vi "read e-series file names.vi"(8 "error in (no error)":errorcluster, 11 "INI File":string) -> (0 "error out":errorcluster, 3 "E-Series File Names":T1)   [LabVIEW 2018, in "E-Series Reader.lvlib"]
doc: "Reads the file names of the E-series from the INI configuration file.\n\nReads an INI configuration file and retrieves the file names associated with the E-series. The VI iterates through the sections defined in the configuration file, retrieves the keys, and reads the value of the <b>Filename</b> key from each section. Returns an array of file names for subsequent loading by <b>Read E Series.vi</b>."
uses:
  E-Series Reader/E-Series Reader.lvlib
  E-Series Reader/E-Series File Names--array.ctl
  <vilib>/Utility/config.llb/Read Key (String).vi
  <vilib>/Utility/config.llb/NI_LVConfig.lvlib
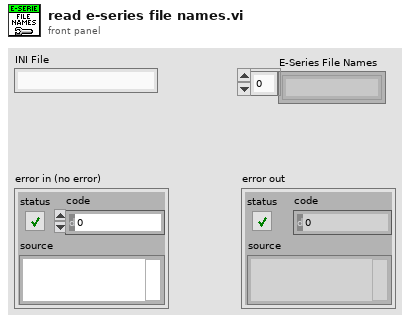
[diagram p1: front panel]
types:
  T1 = typedef "E-Series Reader.lvlib/E-Series File Names--array.ctl" = string[]
  T2 = typedef "NI_LVConfig.lvlib/Config Data RefNum.ctl" = refnum<k1>
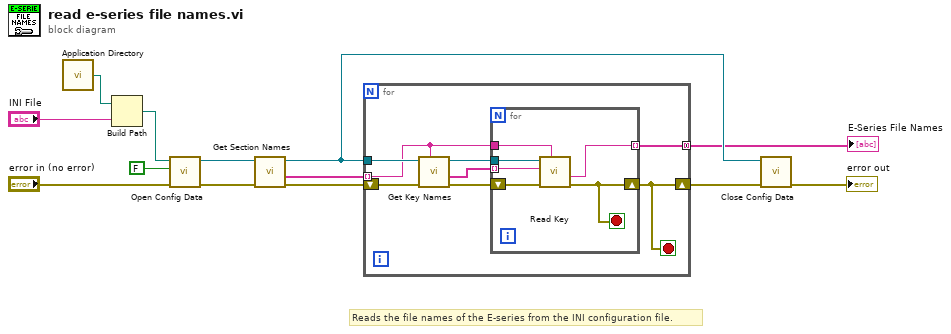
[diagram p0: block diagram]
diagram:
  # "Reads the file names of the E-series from the INI configuration file."
  n1 = call <vilib>:"Application Directory.vi"() -> ("Application Directory"=w12:path)
  n2 = Build Path(base path=w12, name or relative path="INI File") -> (appended path=w10:path)
  n3 = call <vilib>:"Open Config Data.vi"("error in (no error)"="error in (no error)", "create file if necessary (T)"=FALSE, "configuration file path"=w10) -> ("error out"=w9:errorcluster, "refnum"=w7:T2)  [unwired: 6 in, 1 out]
  n4 = call <vilib>:"Get Section Names.vi"("error in (no error)"=w9, "refnum"=w7) -> ("error out"=w8:errorcluster, "section names"=w1:string[], "refnum out"=w4:T2)  [unwired: 7 in]
  n5 = for {
    shift-right: [w14] -> w3
    shift-left: w8 -> [w21]
    tunnel: w1 -> [w18] mode=indexing
    tunnel: w4 -> [w20]
    tunnel: [w16] -> w2 mode=concatenating
    stop <- w14 stop-if-true
    n6 = call <vilib>:"Get Key Names.vi"("section"=w18, "error in (no error)"=w21, "refnum"=w20) -> ("error out"=w19:errorcluster, "key names"=w17:string[], "refnum out"=w15:T2)  [unwired: 5 in, 1 out]
    n7 = for {
      shift-right: [w22] -> w14
      shift-left: w19 -> [w27]
      tunnel: w18 -> [w26]
      tunnel: w17 -> [w25] mode=indexing
      tunnel: [w24] -> w16 mode=indexing
      tunnel: w15 -> [w23]
      stop <- w22 stop-if-true
      n8 = call-poly <vilib>:"Read Key.vi"("section"=w26, "error in (no error)"=w27, "key"=w25, "refnum"=w23) -> ("error out"=w22:errorcluster, "value"=w24:string)  [unwired: 4 in, 2 out]
    }
  }
  "E-Series File Names" <- w2
  n9 = call <vilib>:"Close Config Data.vi"("error in (no error)"=w3, "refnum"=w4) -> ("error out"=→"error out":errorcluster)  [unwired: 8 in, 1 out]
